vi "Create User Event - Stop.vi"(8 "error in (no error)":cluster{"状态":bool, "代码":i32, "源":string} caption="错误输入（无错误）") -> (0 "error out":cluster{"状态":bool, "代码":i32, "源":string} caption="错误输出", 2 "用户事件－停止":refnum<user-event>, 3 "停止事件注册引用句柄":refnum<event-registration>)   [LabVIEW 2018, in "User Event - Stop.lvlib"]
doc: "创建一个布尔用户事件，用于通过“消息处理循环”使“事件循环”停止执行。"
uses:
  User Event - Stop.lvlib
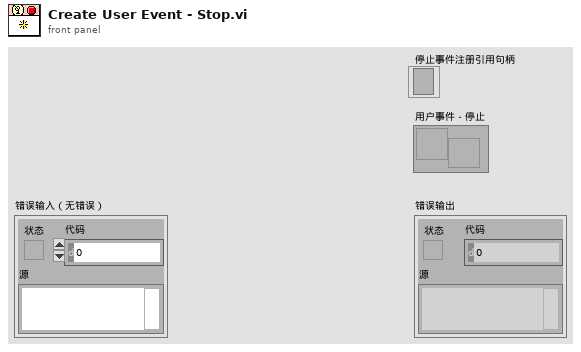
[diagram p1: front panel]
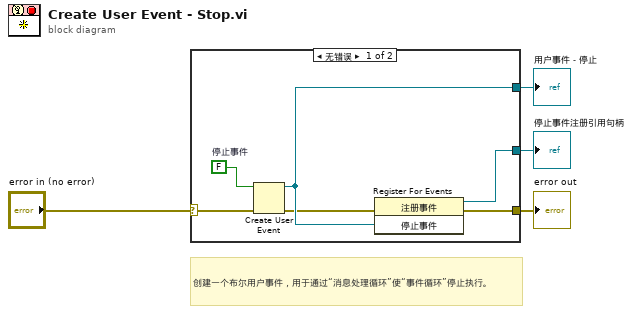
[diagram p0: block diagram]
diagram:
  # "创建一个布尔用户事件，用于通过“消息处理循环”使“事件循环”停止执行。"
  n1 = case shown="无错误" "error in (no error)" {
    selector: "error in (no error)" -> [w5 w11]
    tunnel: [w10 _] -> w4
    tunnel: [w9 _] -> w3
    tunnel: [w6 w11] -> w2
    frame No Error {
      w8 = FALSE  # 停止事件
      n2 = Create User Event(user event datatype=w8, error in=w5) -> (user event=w10:refnum<user-event>, error out=w7:errorcluster)
      n3 = register-events(error in=w7, w10) -> (reference out=w9:refnum<event-registration>, error out=w6:errorcluster)  [unwired: 1 in]
    }
    frame Error {
    }
  }
  "用户事件－停止" <- w4
  "error out" <- w2
  "停止事件注册引用句柄" <- w3
